vi "C(T) data acquisition loop.vi"(0 "Path in":path, 5 "Temp Array In":dbl[](array[numeric]) format="%.2f", 7 "Timing Control Parameters In":T1={"N cycles for averaging"=100, "N points per measurement"=1000, "Measurment time interval"=1e-05} {"Measurment time interval" format="%.2e"}, 11 "error in":errorcluster) -> (4 "Path out":path, 6 "Temp Array Out":dbl[](array[numeric]) format="%.2f", 8 "Timing Control Parameters Out":T1={"N cycles for averaging"=100, "N points per measurement"=1000, "Measurment time interval"=1e-05} {"Measurment time interval" format="%.2e"}, 10 "Normalized Data Out":waveform(dbl)[](array[waveform]), 15 "error out":errorcluster)   [LabVIEW 2016]
doc: "this subvi manages the capacitance measurement cycle\n\nPaul K Dixon\nPhysics 350\nCSUSB Physics"
uses:
  globals/C(T) global variables.vi
panel:
  # "C(T) Acquisition Loop"
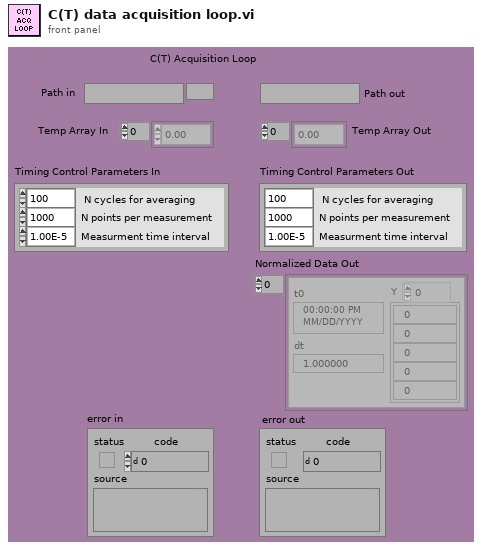
[diagram p1: front panel]
types:
  T1 = cluster{"N cycles for averaging":i32, "N points per measurement":i32, "Measurment time interval":dbl}
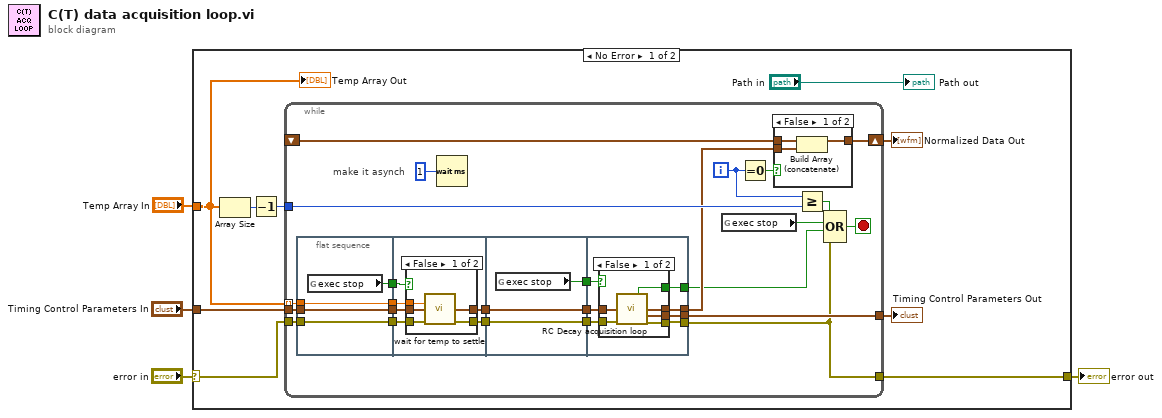
[diagram p0: block diagram]
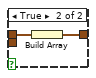
[diagram p4: hidden frame]
diagram:
  n1 = case shown="No Error" "error in" {
    selector: "error in" -> [w6 w79]
    tunnel: "Timing Control Parameters In" -> [w10 _]
    tunnel: [w5 w79] -> w2
    tunnel: "Temp Array In" -> [w7 _]
    frame No Error {
      n2 = Array Size(array=w7) -> (size(s)=w13:i32)
      n3 = Decrement(x=w13) -> (x-1=w12:i32)
      n4 = while {
        tunnel: [w18] -> w9
        shift-left: _ -> [w34]
        shift-right: [w37] -> w11
        tunnel: w12 -> [w38]
        tunnel: w7 -> [w23] mode=indexing
        tunnel: w10 -> [w22]
        tunnel: w6 -> [w16]
        tunnel: [w14] -> w5
        i -> [w36]
        stop <- w31 stop-if-true
        # "make it asynch"
        n5 = flat-sequence {
          tunnel: [w42] -> w29
          tunnel: w23 -> [w41]
          tunnel: w22 -> [w40]
          tunnel: [w41] -> w21
          tunnel: [w40] -> w20
          tunnel: w16 -> [w39]
          tunnel: [w39] -> w15
          tunnel: w29 -> [w48]
          tunnel: [w47] -> w28
          tunnel: [w43] -> w27
          tunnel: w21 -> [w46]
          tunnel: w20 -> [w45]
          tunnel: w15 -> [w44]
          tunnel: [w58] -> w26
          tunnel: w28 -> [w58]
          tunnel: [w57] -> w25
          tunnel: w27 -> [w57]
          tunnel: [w56] -> w24
          tunnel: w26 -> [w65]
          tunnel: w25 -> [w64]
          tunnel: w24 -> [w63]
          tunnel: [w62] -> w19
          tunnel: [w61] -> w18
          tunnel: [w60] -> w14
          tunnel: [w59] -> w17
          frame #0 {
            n6 = global read "C(T) global variables.vi" "exec stop"() -> (w42:bool)
          }
          frame #1 {
            n7 = case shown="False" w48 {
              tunnel: [w52 w55] -> w47
              tunnel: w46 -> [w51 _]
              tunnel: w45 -> [w50 w55]
              tunnel: w44 -> [w49 w54]
              tunnel: [w53 w54] -> w43
              frame False {
                n8 = call "wait for temp to settle.vi"("Current setpoint"=w51, "Timing Control Parameters In"=w50, "error in"=w49) -> ("Timing Control Parameters Out"=w52:T1, "error out"=w53:errorcluster)  [unwired: 2 in, 9 out]
              }
              frame True {
              }
            }
          }
          frame #2 {
            n9 = global read "C(T) global variables.vi" "exec stop"() -> (w56:bool)
          }
          frame #3 {
            n10 = case shown="False" w63 {
              tunnel: [w71 _] -> w59
              tunnel: [w70 w73] -> w60
              tunnel: [w69 _] -> w62
              tunnel: [w68 w72] -> w61
              tunnel: w64 -> [w67 w73]
              tunnel: w65 -> [w66 w72]
              frame False {
                n11 = call "RC Decay acquisition loop.vi"("Timing Control Parameters In"=w66, "error in (no error)"=w67) -> ("time-out?"=w71:bool, "Normalized Waveform Out"=w69:waveform(dbl), "Timing Control Parameters Out"=w68:T1, "error out"=w70:errorcluster)  [unwired: 10 out]
              }
              frame True {
              }
            }
          }
        }
        n12 = Wait (ms)(milliseconds to wait=u32 1) -> ()  [unwired: 1 out]
        n13 = global read "C(T) global variables.vi" "exec stop"() -> (w30:bool)
        n14 = Equal To 0?(x=w36) -> (x = 0?=w35:bool)
        n15 = case shown="False" w35 {
          tunnel: w19 -> [w74 w78]
          tunnel: [w75 w77] -> w37
          tunnel: w34 -> [w76 _]
          frame False {
            n16 = Build Array (concatenate)(w76, w74) -> (w75:waveform(dbl)[])
          }
          frame True {
            n17 = Build Array(w78) -> (w77:waveform(dbl)[])
          }
        }
        n18 = Greater Or Equal?(x=w36, y=w38) -> (x >= y?=w32:bool)
        n19 = Compound Arithmetic op=OR(w32, w30, w17, w14) -> (w31:bool)
      }
      "Normalized Data Out" <- w11
      "Timing Control Parameters Out" <- w9
      "Temp Array Out" <- w7
      "Path out" <- "Path in"
    }
    frame Error {
    }
  }
  "error out" <- w2
